vi "Certificate_03.vi"(0 "CardNumber":string="01:02:03", 2 "DB":T1(ring), 5 "Time":string="12345", 7 "Password":string, 11 "error in":errorcluster) -> (4 "Certificate":u8, 15 "error out":errorcluster)   [LabVIEW 2011]
uses:
  C:/Users/chchung/Desktop/project/Door/DLL/NI.AccessControlSystem.dll
  NI.AccessControlSystem.dll
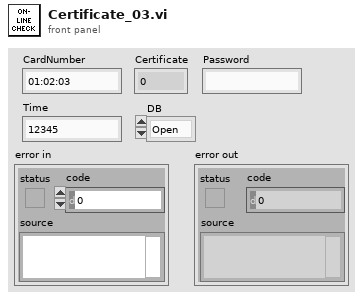
[diagram p1: front panel]
types:
  T1 = enum16{"Open", "Verify", "Password", "Log", "Close"}
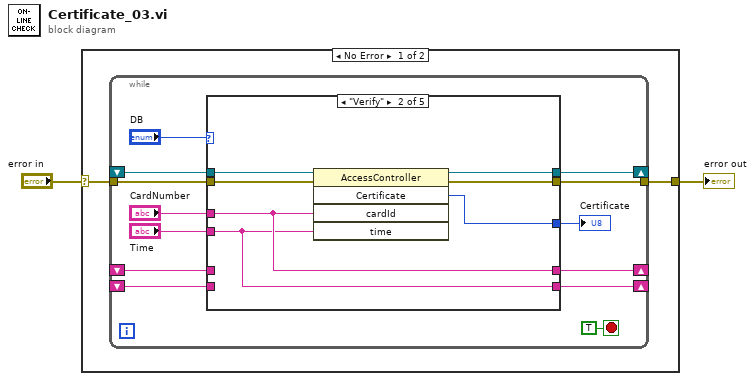
[diagram p0: block diagram]
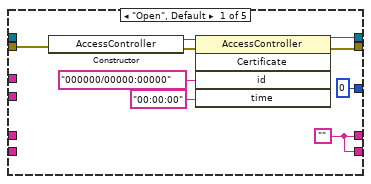
[diagram p2: hidden frame]
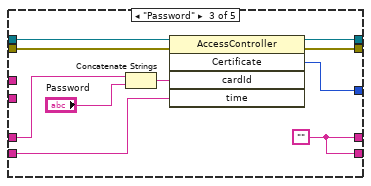
[diagram p3: hidden frame]
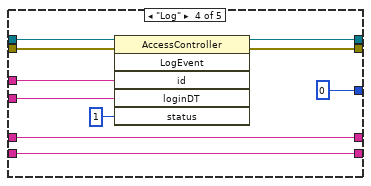
[diagram p4: hidden frame]
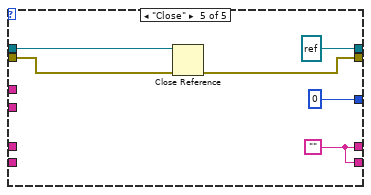
[diagram p5: hidden frame]
diagram:
  n1 = case shown="No Error" "error in" {
    selector: "error in" -> [w4 w60]
    tunnel: [w3 w60] -> w1
    frame No Error {
      n2 = while {
        tunnel: w4 -> [w15]
        tunnel: [w14] -> w3
        shift-right: [w13] -> _
        shift-left: _ -> [w12]
        shift-right: [w8] -> _
        shift-left: _ -> [w6]
        shift-right: [w7] -> _
        shift-left: _ -> [w5]
        stop <- TRUE stop-if-true
        n3 = case shown="\"Verify\"" "DB" {
          tunnel: w15 -> [w26 w33 w43 w52 w59]
          tunnel: [w23 w30 w40 w51 w57] -> w14
          tunnel: [w24 w31 w41 w50 refnum<k24> refnum ("new reference")] -> w13
          tunnel: w12 -> [_ w32 w42 w53 w58]
          tunnel: "CardNumber" -> [_ w28 _ w49 _]
          tunnel: "Time" -> [_ w27 _ w48 _]
          tunnel: [u8 0 ("Certificate") w29 w39 u8 0 ("Certificate") u8 0 ("Certificate")] -> w9
          tunnel: [w19 w28 w37 w46 w54] -> w8
          tunnel: [w19 w27 w37 w45 w54] -> w7
          tunnel: w6 -> [_ _ w36 w46 _]
          tunnel: w5 -> [_ _ w38 w45 _]
          frame "Open", Default {
            w19 = ""
            n4 = constructor class="AccessController"(error in=w26) -> (reference out=w25:refnum<k24>, error out=w22:errorcluster)  [unwired: 2 in, 1 out]
            n5 = invoke class="AccessController" method="Certificate"(reference=w25, error in=w22, "id"="000000/00000:00000", "time"="00:00:00") -> (reference out=w24:refnum<k24>, error out=w23:errorcluster)  [unwired: 1 in, 3 out]
          }
          frame "Verify" {
            n6 = invoke class="AccessController" method="Certificate"(reference=w32, error in=w33, "cardId"=w28, "time"=w27) -> (reference out=w31:refnum<k24>, error out=w30:errorcluster, "Certificate"=w29:u8)  [unwired: 1 in, 2 out]
          }
          frame "Password" {
            w37 = ""
            n7 = Concatenate Strings(w36, "Password") -> (w34:string)
            n8 = invoke class="AccessController" method="Certificate"(reference=w42, error in=w43, "cardId"=w34, "time"=w38) -> (reference out=w41:refnum<k24>, error out=w40:errorcluster, "Certificate"=w39:u8)  [unwired: 1 in, 2 out]
          }
          frame "Log" {
            n9 = invoke class="AccessController" method="LogEvent"(reference=w53, error in=w52, "id"=w49, "loginDT"=w48, "status"=u8 1) -> (reference out=w50:refnum<k24>, error out=w51:errorcluster)  [unwired: 1 in, 4 out]
          }
          frame "Close" {
            w54 = ""
            n10 = Close Reference(reference=w58, error in (no error)=w59) -> (error out=w57:errorcluster)
          }
        }
        "Certificate" <- w9
      }
    }
    frame Error {
    }
  }
  "error out" <- w1
